vi "testWriteFileDefaultEncodingHeaderPresent.vi"(8 "error in (no error)":errorcluster, 11 "TestCase in":refnum<class "EasyXMLTest.lvclass">) -> (0 "error out":errorcluster, 3 "TestCase out":refnum<class "EasyXMLTest.lvclass">)   [LabVIEW 2013, in "EasyXMLTest.lvclass"]
doc: "Verify that no encoding attribute is present if an empty encoding string is specified."
uses:
  EasyXMLTest.lvclass
panel:
  out "XML File Header":string
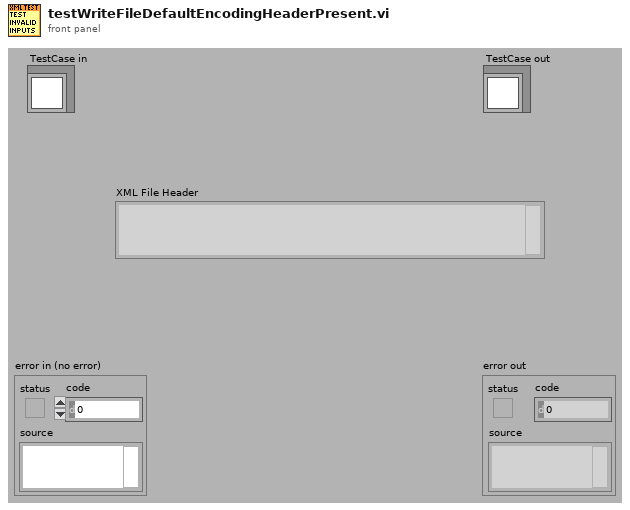
[diagram p1: front panel]
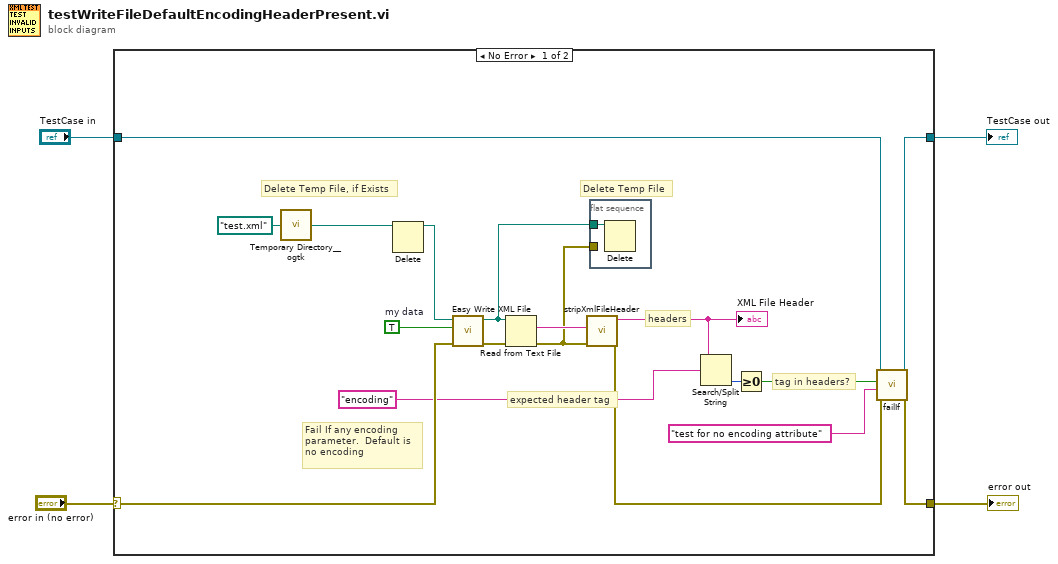
[diagram p0: block diagram]
diagram:
  n1 = case shown="No Error" "error in (no error)" {
    selector: "error in (no error)" -> [w21 w25]
    tunnel: [w8 w25] -> w3
    tunnel: [w10 w24] -> w1
    tunnel: "TestCase in" -> [w11 w24]
    frame No Error {
      w22 = TRUE  # my data
      # "Fail If any encoding parameter.  Default is no encoding"
      # "tag in headers?"
      # "headers"
      # "expected header tag"
      # "Delete Temp File"
      # "Delete Temp File, if Exists"
      n2 = call <userlib>:"Temporary Directory__ogtk.vi"("Relative path (.)"=path "test.xml") -> ("Temporary Directory (+ Relative)"=w19:path)
      n3 = Delete(path (use dialog)=w19) -> (deleted path=w18:path)  [unwired: 4 in, 2 out]
      n4 = call "Easy Write XML File.vi"("error in (no error)"=w21, "LabVIEW Data"=w22, "XML File Path"=w18) -> ("error out"=w16:errorcluster, "XML File Path (duplicate)"=w17:path)  [unwired: 7 in]
      n5 = Read from Text File(file (use dialog)=w17, error in=w16) -> (text=w15:string, error out=w14:errorcluster)  [unwired: 2 in, 2 out]
      n6 = call "stripXmlFileHeader.vi"("error in (no error)"=w14, "XML File String"=w15) -> ("error out"=w9:errorcluster, "XML File Header"=w13:string)  [unwired: 7 in, 1 out]
      "XML File Header" <- w13
      n7 = flat-sequence {
        tunnel: w17 -> [w23]
        tunnel: w14 -> [_]
        frame #0 {
          n8 = Delete(path (use dialog)=w23) -> ()  [unwired: 4 in, 3 out]
        }
      }
      n9 = Search/Split String(string=w13, search string/char (-)="encoding") -> (offset of match=w12:i32)  [unwired: 1 in, 2 out]
      n10 = Greater Or Equal To 0?(x=w12) -> (x >= 0?=w7:bool)
      n11 = call-dynamic "failIf.vi"("error in (no error)"=w9, "message (\"\")"="test for no encoding attribute" ("message (\"\")"), "fail"=w7, "TestCase in"=w11) -> ("error out"=w8:errorcluster, "TestCase out"=w10:refnum<class "EasyXMLTest.lvclass">)  [unwired: 6 in]
    }
    frame Error {
    }
  }
  "error out" <- w3
  "TestCase out" <- w1
